vi "StartCam.vi"(8 "error in":errorcluster, 11 "Session In":T2) -> (0 "error out":errorcluster, 2 "New Image":T1, 3 "Session Out":T2)   [LabVIEW 2018]
uses:
  <vilib>/userdefined/High Color/IMAQdx.ctl
  <vilib>/vision/Image Controls.llb/IMAQ Image.ctl
  <vilib>/vision/driver/NI_Vision_Acquisition_Software.lvlib
  <resource>/objmgr/imaqdx.rc
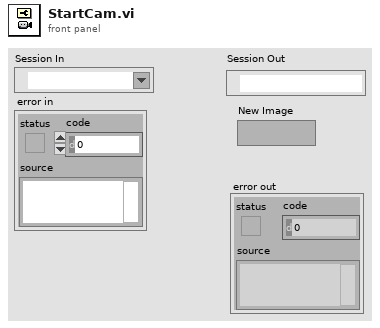
[diagram p1: front panel]
types:
  T1 = typedef "IMAQ Image.ctl" = refnum<image>
  T2 = typedef "IMAQdx.ctl" = refnum<k21>
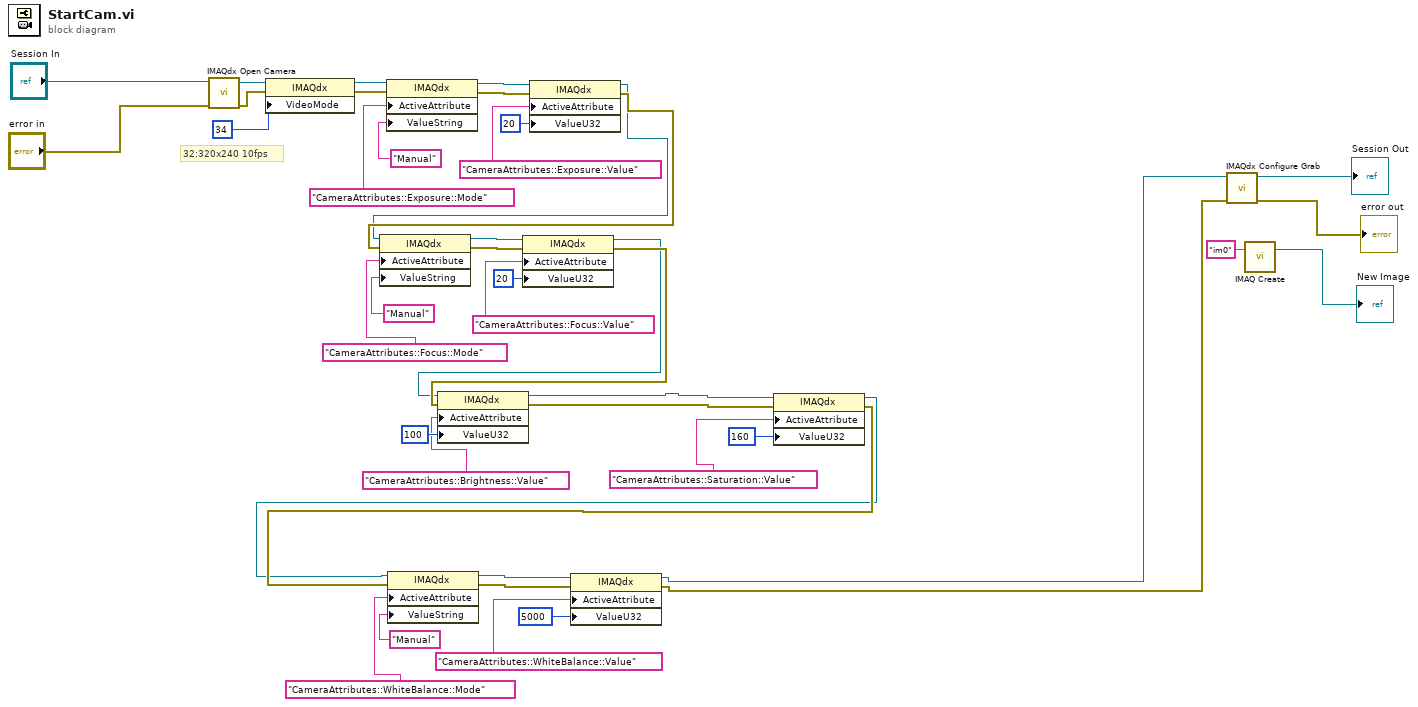
[diagram p0: block diagram]
diagram:
  # "32:320x240 10fps"
  n1 = call <vilib>:"IMAQdx Open Camera.vi"("error in"="error in", "Session In"="Session In") -> ("error out"=w21:errorcluster, "Session Out"=w22:T2)  [unwired: 8 in]
  n2 = property class="IMAQdx"(reference=w22, error in=w21, "VideoMode"=u32 34) -> (reference out=w23:T2, error out=w24:errorcluster)
  n3 = property class="IMAQdx"(reference=w23, error in=w24, "ActiveAttribute"="CameraAttributes::Exposure::Mode", "ValueString"="Manual") -> (reference out=w27:T2, error out=w28:errorcluster)
  n4 = property class="IMAQdx"(reference=w27, error in=w28, "ActiveAttribute"="CameraAttributes::Exposure::Value", "ValueU32"=u32 20) -> (reference out=w39:T2, error out=w40:errorcluster)
  n5 = property class="IMAQdx"(reference=w39, error in=w40, "ActiveAttribute"="CameraAttributes::Focus::Mode", "ValueString"="Manual") -> (reference out=w34:T2, error out=w33:errorcluster)
  n6 = property class="IMAQdx"(reference=w34, error in=w33, "ActiveAttribute"="CameraAttributes::Focus::Value", "ValueU32"=u32 20) -> (reference out=w41:T2, error out=w42:errorcluster)
  n7 = property class="IMAQdx"(reference=w41, error in=w42, "ActiveAttribute"="CameraAttributes::Brightness::Value", "ValueU32"=u32 100) -> (reference out=w5:T2, error out=w4:errorcluster)
  n8 = property class="IMAQdx"(reference=w5, error in=w4, "ActiveAttribute"="CameraAttributes::Saturation::Value", "ValueU32"=u32 160) -> (reference out=w2:T2, error out=w3:errorcluster)
  n9 = property class="IMAQdx"(reference=w2, error in=w3, "ActiveAttribute"="CameraAttributes::WhiteBalance::Mode", "ValueString"="Manual") -> (reference out=w11:T2, error out=w12:errorcluster)
  n10 = property class="IMAQdx"(reference=w11, error in=w12, "ActiveAttribute"="CameraAttributes::WhiteBalance::Value", "ValueU32"=u32 5000) -> (reference out=w8:T2, error out=w7:errorcluster)
  n11 = call <vilib>:"IMAQdx Configure Grab.vi"("error in"=w7, "Session In"=w8) -> ("error out"=→"error out":errorcluster, "Session Out"=→"Session Out":T2)  [unwired: 8 in]
  n12 = call "IMAQ Create"("Image Name"="im0") -> ("New Image"=→"New Image":T1)  [unwired: 4 in, 1 out]
